vi "deserializeMissionArray.vi"(8 "Error In":errorcluster, 11 "Serialized Mission Array":string) -> (0 "Error Out":errorcluster, 3 "Mission Object Array":refnum<class "GenericMission.lvclass">[](array[class]))   [LabVIEW 2011]
uses:
  GenericMission/GenericMission.lvclass
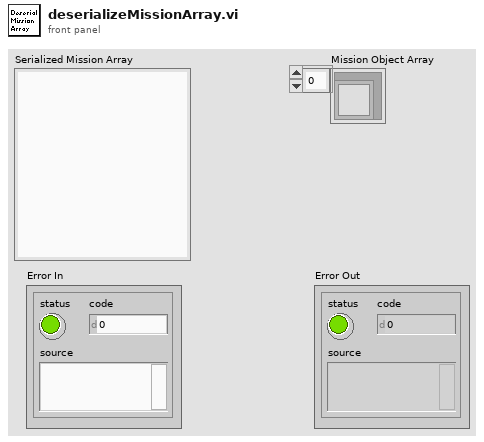
[diagram p1: front panel]
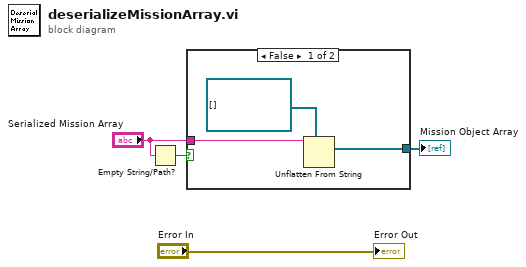
[diagram p0: block diagram]
diagram:
  n1 = Empty String/Path?(string/path="Serialized Mission Array") -> (empty?=w3:bool)
  n2 = case shown="False" w3 {
    tunnel: [w6 _] -> w2
    tunnel: "Serialized Mission Array" -> [w7 _]
    frame False {
      n3 = Unflatten From String(type=refnum<class "GenericMission.lvclass">[] [] ("Mission Object Array"), binary string=w7) -> (value=w6:refnum<class "GenericMission.lvclass">[])  [unwired: 3 in, 2 out]
    }
    frame True {
    }
  }
  "Mission Object Array" <- w2
  "Error Out" <- "Error In"
